vi "ad get samples.vi"(0 "adh":i32, 1 "n":u32, 5 "index":i32, 7 "type":i32, 9 "offset":dbl, 11 "error in (no error)":errorcluster, 12 "buf":u32) -> (3 "n out":u32, 4 "function return":i32, 14 "buf out":u32, 15 "error out":errorcluster)   [LabVIEW 2021, in "libad4.lvlib"]
doc: "LIBAD4 function: ad_get_samples (int32_t adh, int32_t index, int32_t type, uint64_t offset, uint32_t *n, void *buf);\n\nReads samples from the scan buffer. Requires AD_SF_SAMPLES flag to be set."
uses:
  <userlib>/libad4/libad4.lvlib
  <userlib>/libad4/libad4.dll
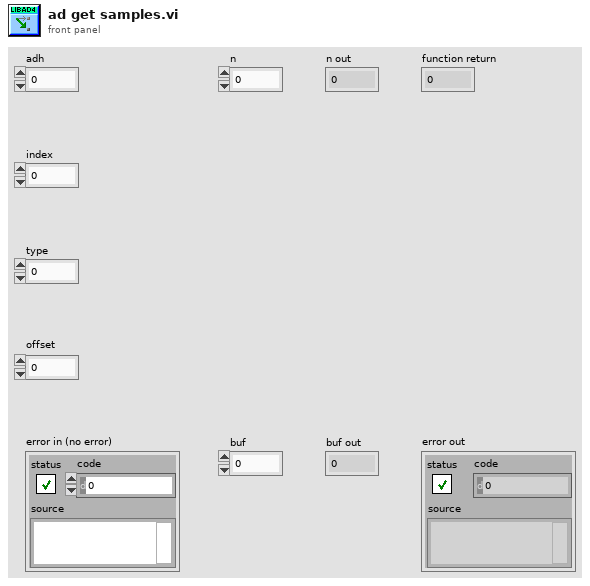
[diagram p1: front panel]
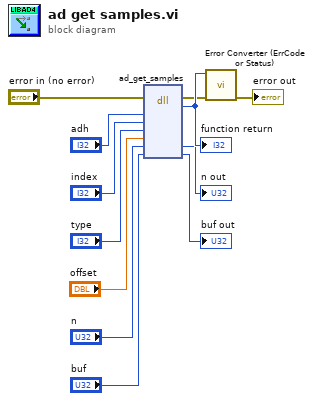
[diagram p0: block diagram]
diagram:
  n1 = dll-call lib="C:/Program Files/National Instruments/LabVIEW 2021/user.lib/libad4/libad4.*" fn="ad_get_samples"(error in="error in (no error)", "adh"="adh", "index"="index", "type"="type", "offset"="offset", "n"="n", "buf"="buf") -> (error out=w2:errorcluster, w12:i32, "n"=→"n out":u32, "buf"=→"buf out":u32)  [unwired: 6 in, 1 out]
  "function return" <- w12
  n2 = call <userlib>:"Error Converter (ErrCode or Status).vi"("error in (no error)"=w2, "error code"=w12) -> ("error out"=→"error out":errorcluster)  [unwired: 9 in]
